vi "RFmx_Meas_Fetch_Results.vi"(8 "error in":errorcluster, 10 "Measurements":T1(array[ring]), 11 "Instrument Handle in":refnum<k21>) -> (0 "error out":errorcluster, 3 "Instrument Handle out":refnum<k21>)   [LabVIEW 2014]
uses:
  <vilib>/RFmx/SpecAn/mx/RFmxSpecAn.llb/RFmxSpecAn ACP Fetch Total Carrier Power.vi
  <vilib>/RFmx/SpecAn/mx/RFmxSpecAn.llb/RFmxSpecAn ACP Fetch Offset Measurement (Array).vi
  <vilib>/RFmx/SpecAn/mx/RFmxSpecAn.llb/RFmxSpecAn CCDF Fetch Power.vi
  <vilib>/RFmx/SpecAn/mx/RFmxSpecAn.llb/RFmxSpecAn CHP Fetch Total Carrier Power.vi
  <vilib>/RFmx/SpecAn/mx/RFmxSpecAn.llb/RFmxSpecAn FCnt Fetch Measurement.vi
  <vilib>/RFmx/SpecAn/mx/RFmxSpecAn.llb/RFmxSpecAn OBW Fetch Measurement.vi
  <vilib>/RFmx/SpecAn/mx/RFmxSpecAn.llb/RFmxSpecAn Spectrum Fetch Measurement.vi
  <vilib>/RFmx/SpecAn/mx/RFmxSpecAn.llb/RFmxSpecAn TXP Fetch Measurement.vi
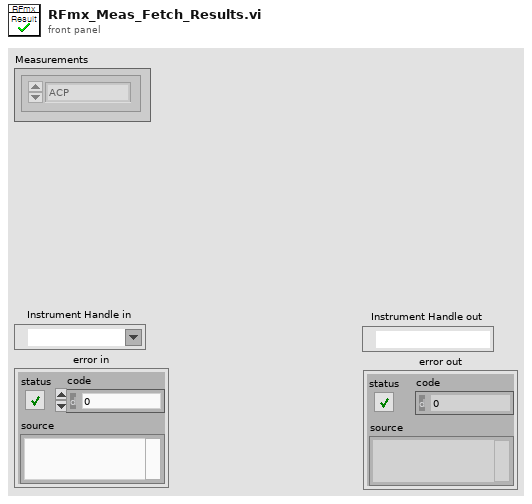
[diagram p1: front panel]
types:
  T1 = enum16{"ACP", "CCDF", "CHP", "FCnt", "Harmonics", "OBW", "SEM", "Spectrum", "Spur", "TXP", "AMPM", "DPD", "IQ"}[]
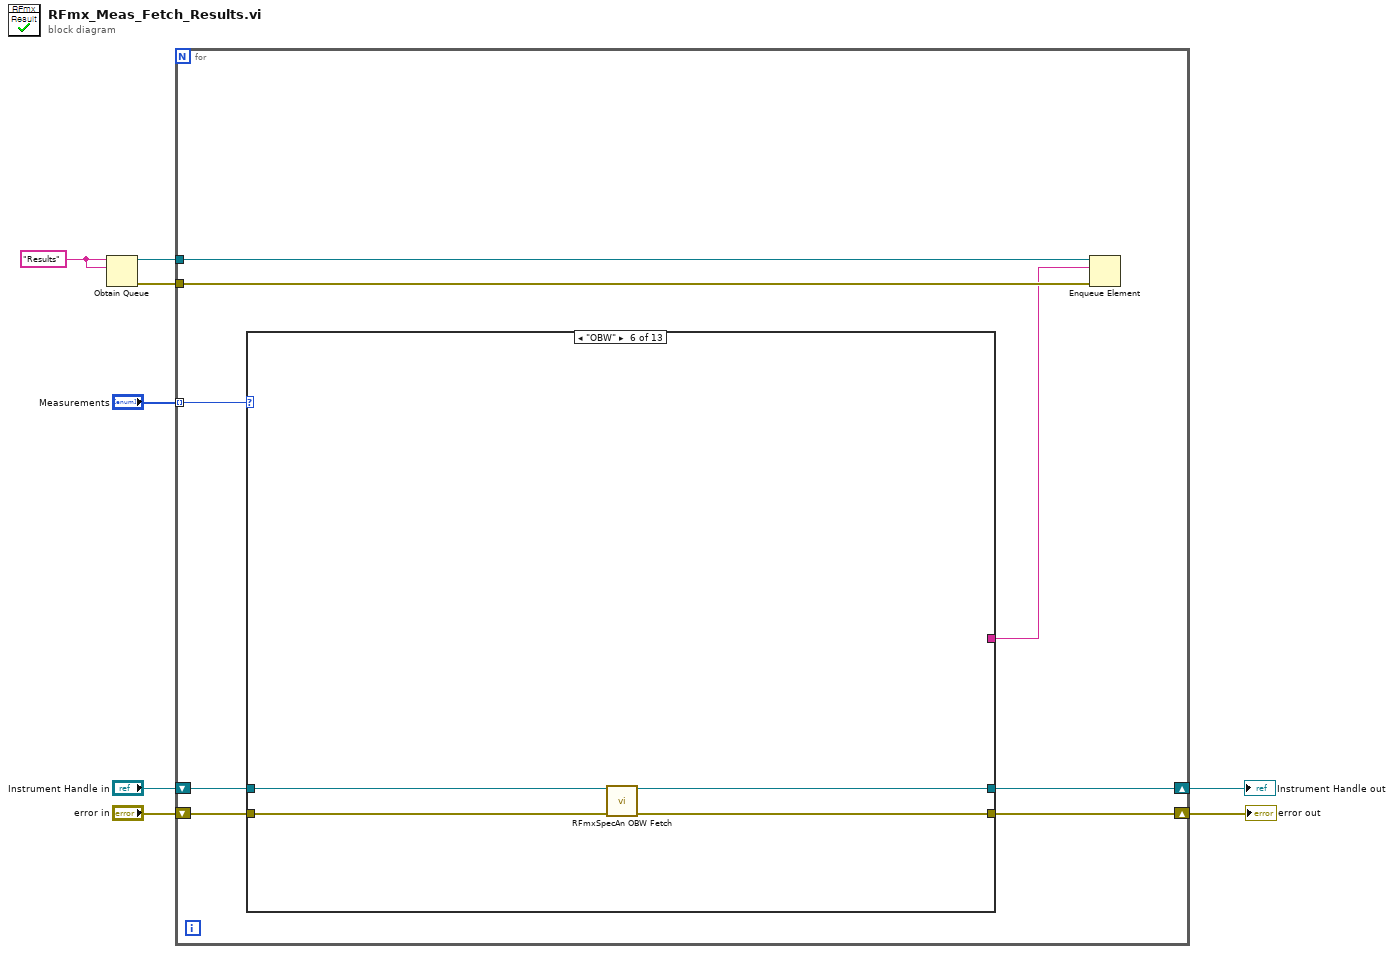
[diagram p0: block diagram]
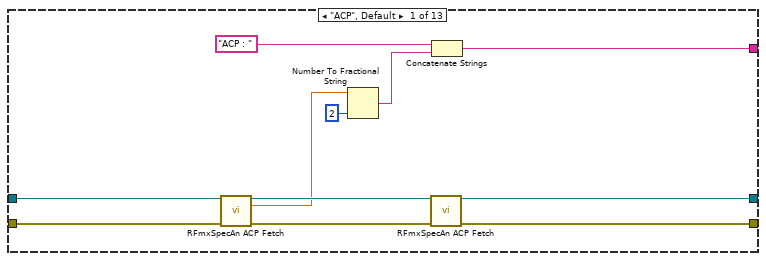
[diagram p2: hidden frame]
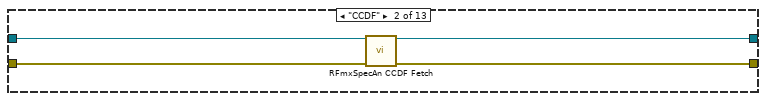
[diagram p3: hidden frame]
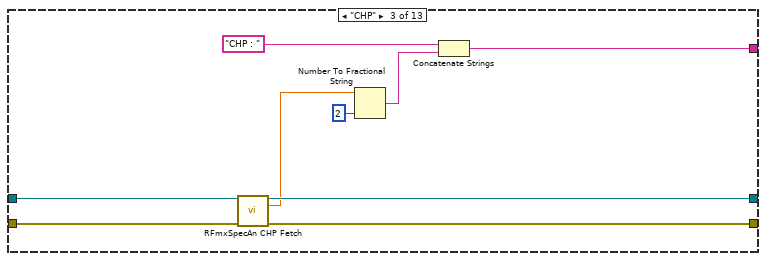
[diagram p4: hidden frame]
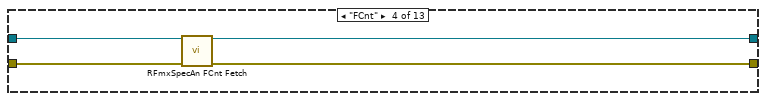
[diagram p5: hidden frame]
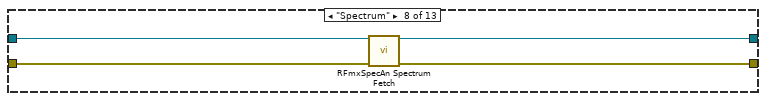
[diagram p8: hidden frame]
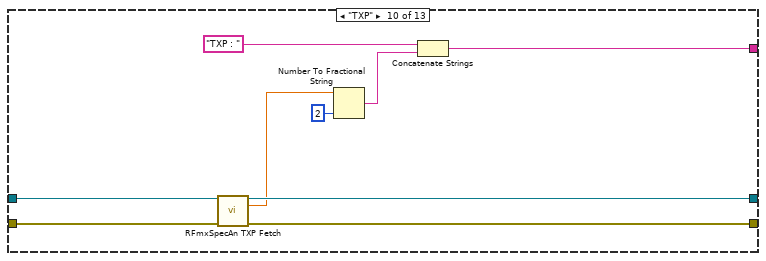
[diagram p10: hidden frame]
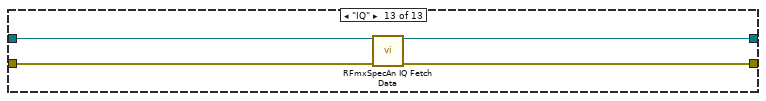
[diagram p13: hidden frame]
diagram:
  w3 = "Results" ("name (unnamed)")
  n1 = Obtain Queue(name (unnamed)=w3, element data type=w3) -> (queue out=w2:refnum<queue>, error out=w1:errorcluster)  [unwired: 3 in, 1 out]
  n2 = for {
    shift-right: [w16] -> w8
    shift-left: "Instrument Handle in" -> [w13]
    shift-right: [w15] -> w7
    shift-left: "error in" -> [w12]
    tunnel: "Measurements" -> [w14] mode=indexing
    tunnel: w2 -> [w11]
    tunnel: w1 -> [w10]
    n3 = case shown="\"OBW\"" w14 {
      tunnel: w13 -> [w27 w31 w40 w44 w45 w50 w52 w56 w58 w67 w69 w71 w75]
      tunnel: w12 -> [w26 w30 w39 w43 w46 w49 w51 w55 w57 w66 w68 w70 w74]
      tunnel: [w23 w29 w38 w42 w45 w48 w52 w53 w58 w65 w69 w71 w72] -> w16
      tunnel: [w22 w28 w37 w41 w46 w47 w51 w54 w57 w64 w68 w70 w73] -> w15
      tunnel: [w17 _ w32 _ _ _ _ _ _ w59 _ _ _] -> w9
      frame "ACP", Default {
        n4 = call-poly <vilib>:"RFmxSpecAn ACP Fetch.vi"("Instrument Handle In"=w27, "error in (no error)"=w26) -> ("Instrument Handle Out"=w25:refnum<k21>, "Total Carrier Power (dBm or dBm/Hz)"=w21:dbl, "error out"=w24:errorcluster)  [unwired: 11 in]
        n5 = Number To Fractional String(number=w21, precision (6)=i16 2) -> (F-format string=w18:string)  [unwired: 2 in]
        n6 = call-poly <vilib>:"RFmxSpecAn ACP Fetch.vi"("Instrument Handle In"=w25, "error in (no error)"=w24) -> ("Instrument Handle Out"=w23:refnum<k21>, "error out"=w22:errorcluster)  [unwired: 8 in, 4 out]
        n7 = Concatenate Strings("ACP : " ("name (unnamed)"), w18) -> (w17:string)
      }
      frame "CCDF" {
        n8 = call-poly <vilib>:"RFmxSpecAn CCDF Fetch.vi"("Instrument Handle In"=w31, "error in (no error)"=w30) -> ("Instrument Handle Out"=w29:refnum<k21>, "error out"=w28:errorcluster)  [unwired: 8 in, 4 out]
      }
      frame "CHP" {
        n9 = call-poly <vilib>:"RFmxSpecAn CHP Fetch.vi"("Instrument Handle In"=w40, "error in (no error)"=w39) -> ("Instrument Handle Out"=w38:refnum<k21>, "Total Carrier Power (dBm)"=w33:dbl, "error out"=w37:errorcluster)  [unwired: 11 in]
        n10 = Number To Fractional String(number=w33, precision (6)=i16 2) -> (F-format string=w34:string)  [unwired: 2 in]
        n11 = Concatenate Strings("CHP : " ("name (unnamed)"), w34) -> (w32:string)
      }
      frame "FCnt" {
        n12 = call-poly <vilib>:"RFmxSpecAn FCnt Fetch.vi"("Instrument Handle In"=w44, "error in (no error)"=w43) -> ("Instrument Handle Out"=w42:refnum<k21>, "error out"=w41:errorcluster)  [unwired: 9 in, 3 out]
      }
      frame "Harmonics" {
        # "Harmonics는 5665, 5668R에만 적용 가능함"
      }
      frame "OBW" {
        n13 = call-poly <vilib>:"RFmxSpecAn OBW Fetch.vi"("Instrument Handle In"=w50, "error in (no error)"=w49) -> ("Instrument Handle Out"=w48:refnum<k21>, "error out"=w47:errorcluster)  [unwired: 7 in, 5 out]
      }
      frame "SEM" {
        # "적용해야할 부분이 많으므로 다음에 추가할 예정"
      }
      frame "Spectrum" {
        n14 = call-poly <vilib>:"RFmxSpecAn Spectrum Fetch.vi"("Instrument Handle In"=w56, "error in (no error)"=w55) -> ("Instrument Handle Out"=w53:refnum<k21>, "error out"=w54:errorcluster)  [unwired: 9 in, 3 out]
      }
      frame "Spur" {
        # "Spur는 5665, 5668R에만 적용 가능함"
      }
      frame "TXP" {
        n15 = call-poly <vilib>:"RFmxSpecAn TXP Fetch.vi"("Instrument Handle In"=w67, "error in (no error)"=w66) -> ("Instrument Handle Out"=w65:refnum<k21>, "Average Mean Power (dBm)"=w60:dbl, "error out"=w64:errorcluster)  [unwired: 8 in, 3 out]
        n16 = Number To Fractional String(number=w60, precision (6)=i16 2) -> (F-format string=w61:string)  [unwired: 2 in]
        n17 = Concatenate Strings("TXP : " ("name (unnamed)"), w61) -> (w59:string)
      }
      frame "AMPM" {
        # "적용해야할 부분이 많으므로 다음에 추가할 예정"
      }
      frame "DPD" {
        # "적용해야할 부분이 많으므로 다음에 추가할 예정"
      }
      frame "IQ" {
        n18 = call <vilib>:"RFmxSpecAn IQ Fetch Data.vi"("Instrument Handle In"=w75, "error in (no error)"=w74) -> ("Instrument Handle Out"=w72:refnum<k21>, "error out"=w73:errorcluster)  [unwired: 11 in, 1 out]
      }
    }
    n19 = Enqueue Element(queue=w11, element=w9, error in (no error)=w10) -> ()  [unwired: 1 in, 3 out]
  }
  "Instrument Handle out" <- w8
  "error out" <- w7
